vi "ubinary_load.vi"(8 "error in":errorcluster, 9 "control":string, 10 "file (use dialog)":path, 11 "VI":refnum<vi>) -> (0 "error out":errorcluster)   [LabVIEW 2012]
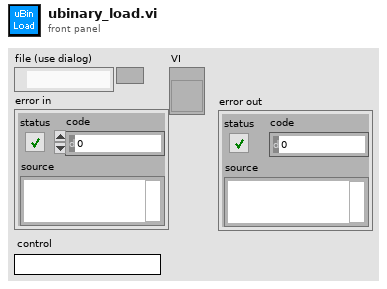
[diagram p1: front panel]
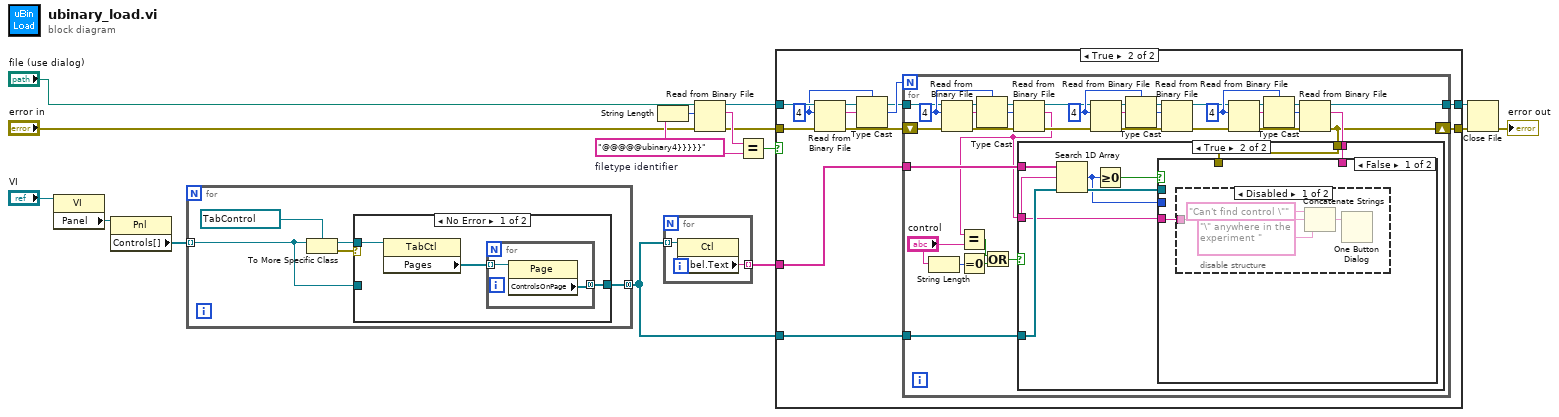
[diagram p0: block diagram]
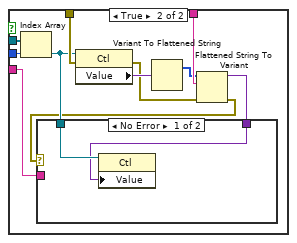
[diagram p5: hidden frame]
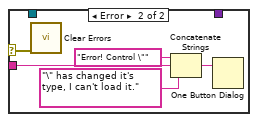
[diagram p6: hidden frame]
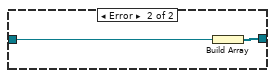
[diagram p7: hidden frame]
diagram:
  w11 = "@@@@@ubinary4}}}}}"  # filetype identifier
  n1 = property class="VI"(reference="VI") -> ("Panel"=w16:refnum<vi>)  [unwired: 1 in, 2 out]
  n2 = property class="Pnl"(reference=w16) -> ("Controls[]"=w15:refnum<vi>[])  [unwired: 1 in, 2 out]
  n3 = for {
    tunnel: w15 -> [w18] mode=indexing
    tunnel: [w17] -> w1 mode=concatenating
    n4 = To More Specific Class(target class=refnum<vi> refnum ("reference"), reference=w18) -> (specific class reference=w20:refnum<vi>, error out=w19:errorcluster)  [unwired: 1 in]
    n5 = case shown="No Error" w19 {
      tunnel: w20 -> [w24 _]
      tunnel: [w22 w28] -> w17
      tunnel: w18 -> [_ w27]
      frame No Error {
        n6 = property on="Property Node" class="TabCtl"(reference=w24) -> ("Pages"=w23:refnum<vi>[])  [unwired: 1 in, 2 out]
        n7 = for {
          tunnel: w23 -> [w26] mode=indexing
          tunnel: [w25] -> w22 mode=concatenating
          n8 = property class="Page"(reference=w26) -> ("ControlsOnPage"=w25:refnum<vi>[])  [unwired: 1 in, 2 out]
        }
      }
      frame Error {
        n9 = Build Array(w27) -> (w28:refnum<vi>[])
      }
    }
  }
  n10 = String Length(string=w11) -> (length=w12:i32)
  n11 = for {
    tunnel: w1 -> [w30] mode=indexing
    tunnel: [w29] -> w6 mode=indexing
    n12 = property class="Ctl"(reference=w30) -> ("Label.Text"=w29:string)  [unwired: 1 in, 2 out]
  }
  n13 = Read from Binary File(8:"error in", 10:w12, 11:"file (use dialog)") -> (0:w7:errorcluster, 2:w10:string, 3:w9:refnum<file>)  [unwired: 3 in, 1 out]
  n14 = Equal?(x=w10, y=w11) -> (x = y?=w8:bool)
  n15 = case shown="True" w8 {
    tunnel: [w32 w33] -> w13
    tunnel: w9 -> [w32 w43]
    tunnel: w7 -> [w31 w38]
    tunnel: w6 -> [_ w37]
    tunnel: [w31 w36] -> w5
    tunnel: w1 -> [_ w35]
    frame False {
    }
    frame True {
      w41 = 4 ("count (1)")
      n16 = Read from Binary File(8:w38, 10:w41, 11:w43) -> (0:w39:errorcluster, 2:w42:string, 3:w34:refnum<file>)  [unwired: 3 in, 1 out]
      n17 = Type Cast(type=w41, x=w42) -> (*(type *) &x=w40:i32)
      n18 = for {
        N: w40 -> [_]
        tunnel: w34 -> [w73]
        shift-right: [w50] -> w36
        shift-left: w39 -> [w69]
        tunnel: w37 -> [w68]
        tunnel: w35 -> [w53]
        tunnel: [w51] -> w33
        w62 = 4 ("count (1)")
        w63 = 4 ("count (1)")
        w75 = 4 ("count (1)")
        n19 = String Length(string="control") -> (length=w46:i32)
        n20 = Read from Binary File(8:w69, 10:w75, 11:w73) -> (0:w70:errorcluster, 2:w74:string, 3:w72:refnum<file>)  [unwired: 3 in, 1 out]
        n21 = Equal To 0?(x=w46) -> (x = 0?=w45:bool)
        n22 = Type Cast(type=w75, x=w74) -> (*(type *) &x=w71:i32)
        n23 = Read from Binary File(8:w70, 10:w71, 11:w72) -> (0:w56:errorcluster, 2:w49:string, 3:w57:refnum<file>)  [unwired: 3 in, 1 out]
        n24 = Equal?(x=w49, y="control") -> (x = y?=w47:bool)
        n25 = Or(x=w47, y=w45) -> (x .or. y?=w48:bool)
        n26 = Read from Binary File(8:w56, 10:w63, 11:w57) -> (0:w67:errorcluster, 2:w64:string, 3:w65:refnum<file>)  [unwired: 3 in, 1 out]
        n27 = Type Cast(type=w63, x=w64) -> (*(type *) &x=w66:i32)
        n28 = Read from Binary File(8:w67, 10:w66, 11:w65) -> (0:w55:errorcluster, 3:w54:refnum<file>)  [unwired: 3 in, 2 out]
        n29 = Read from Binary File(8:w55, 10:w62, 11:w54) -> (0:w58:errorcluster, 2:w61:string, 3:w60:refnum<file>)  [unwired: 3 in, 1 out]
        n30 = Type Cast(type=w62, x=w61) -> (*(type *) &x=w59:i32)
        n31 = Read from Binary File(8:w58, 10:w59, 11:w60) -> (0:w50:errorcluster, 2:w52:string, 3:w51:refnum<file>)  [unwired: 3 in, 1 out]
        n32 = case shown="True" w48 {
          tunnel: w68 -> [_ w82]
          tunnel: w53 -> [_ w80]
          tunnel: w52 -> [_ w78]
          tunnel: w49 -> [_ w77]
          tunnel: w50 -> [_ w76]
          frame False {
          }
          frame True {
            n33 = Search 1D Array(1D array=w82, element=w77) -> (index of element=w79:i32)  [unwired: 1 in]
            n34 = Greater Or Equal To 0?(x=w79) -> (x >= 0?=w81:bool)
            n35 = case shown="False" w81 {
              tunnel: w80 -> [_ w98]
              tunnel: w79 -> [_ w97]
              tunnel: w78 -> [_ w96]
              tunnel: w77 -> [w83 w88]
              tunnel: w76 -> [_ w92]
              frame False {
                n36 = disable-structure shown="Disabled" {
                  disable-tunnel: w83 -> [w87 _]
                  frame Disabled {
                    n37 = Concatenate Strings("Can't find control \"" ("string"), w87, "\" anywhere in the experiment " ("string")) -> (w86:string)
                    n38 = One Button Dialog(message=w86) -> ()  [unwired: 1 in, 1 out]
                  }
                  frame Enabled {
                  }
                }
              }
              frame True {
                n39 = Index Array(array=w98, index=w97) -> (element=w91:refnum<vi>)
                n40 = property class="Ctl"(reference=w91, error in=w92) -> (error out=w93:errorcluster, "Value"=w95:variant)  [unwired: 1 out]
                n41 = Variant To Flattened String(Variant=w95) -> (1:w94:i16[])  [unwired: 1 out]
                n42 = Flattened String To Variant(4:w93, 6:w96, 7:w94) -> (0:w90:errorcluster, 3:w89:variant)
                n43 = case shown="No Error" w90 {
                  selector: w90 -> [_ w105]
                  tunnel: w91 -> [w100 _]
                  tunnel: w89 -> [w99 _]
                  tunnel: w88 -> [_ w103]
                  frame No Error {
                    n44 = property class="Ctl"(reference=w100, "Value"=w99) -> ()  [unwired: 1 in, 2 out]
                  }
                  frame Error {
                    n45 = call <vilib>:"Clear Errors.vi"("error in (no error)"=w105) -> ()  [unwired: 6 in, 1 out]
                    n46 = Concatenate Strings("Error! Control \"" ("string"), w103, "\" has changed it's type, I can't load it." ("string")) -> (w104:string)
                    n47 = One Button Dialog(message=w104) -> ()  [unwired: 1 in, 1 out]
                  }
                }
              }
            }
          }
        }
      }
    }
  }
  n48 = Close File(refnum=w13, error in=w5) -> (error out=→"error out":errorcluster)  [unwired: 1 out]
